vi "Init Error Window.vi"(4 "Window Vertical Size (pixels)":i16=600, 5 "Window Behaviour":T1, 6 "Window Horizontal Size (pixels)":i16=800, 7 "Window Close (X) Button Enabled? (Default = True)":bool=TRUE, 8 "Error In":errorcluster, 9 "Background Colour (Default = 255,255,255)":u32(colorbox)=16777215, 10 "Window Title":string="Modal Dialogue", 11 "VI Refnum":refnum<vi>) -> (0 "Error Out":errorcluster)   [LabVIEW 2016, in "Error Manager.lvlib"]
doc: "This VI configures the Front Panel (the GUI Window) of the VI whose refnum is passed as an argument to the \"VI Refnum\" input (usually, the immediate caller VI)."
uses:
  Error Manager.lvlib
  <vilib>/Utility/miscctls.llb/LVPointTypeDef.ctl
  <vilib>/Utility/miscctls.llb/LVRectTypeDef.ctl
  Settings/Window_Behaviour (enum).ctl
  Settings/Settings.lvclass
panel:
  # "Development\ncontrols/indicators useful for development and testing, but which are not outputs of the VI"
  # "Input\nInputs to the VI"
  # "Output\nOutputs of the VI"
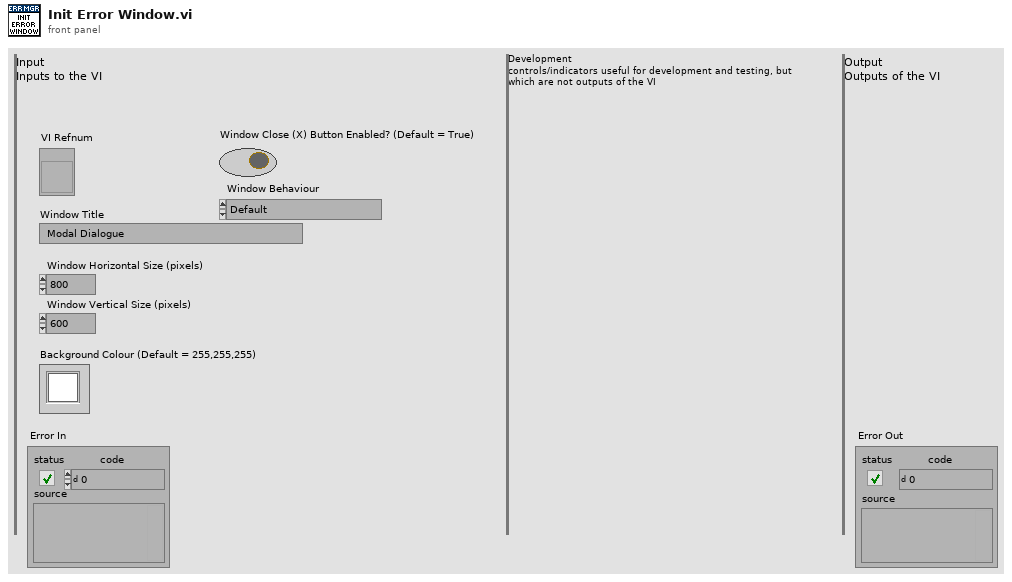
[diagram p1: front panel]
types:
  T1 = typedef "Error Manager.lvlib/Settings.lvclass/Window_Behaviour (enum).ctl" = enum16{"Default", "Floating", "Modal"}
  T2 = enum32{"Invalid", "Standard", "Closed", "Hidden", "Minimized", "Maximized"}
  T3 = typedef "LVRectTypeDef.ctl" = cluster{"Left":i16, "Top":i16, "Right":i16, "Bottom":i16}
  T4 = typedef "LVPointTypeDef.ctl" = cluster{"Horizontal":i16, "Vertical":i16}
  T5 = enum16{"Always On", "Always Off", "Off While Running"}
  T6 = enum32{"Invalid", "Default", "Floating", "Floating/Auto-Hide", "Modal"}
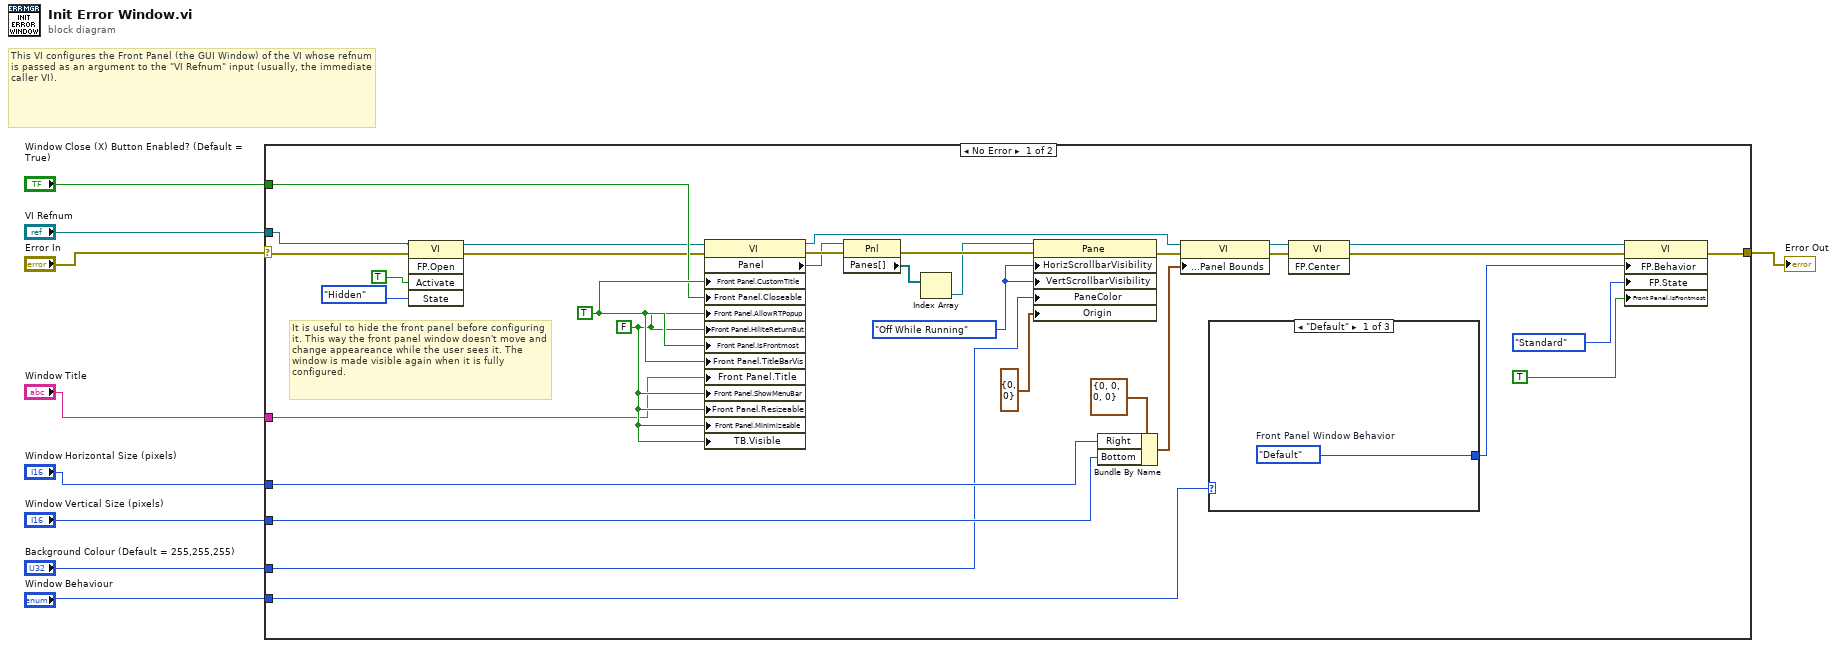
[diagram p0: block diagram]
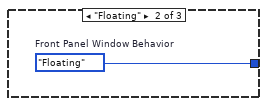
[diagram p2: hidden frame]
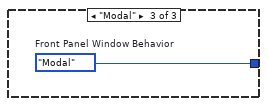
[diagram p3: hidden frame]
diagram:
  # "This VI configures the Front Panel (the GUI Window) of the VI whose refnum is passed as an argument to the \"VI Refnum\" input (usually, the immediate caller VI)."
  n1 = case shown="No Error" "Error In" {
    selector: "Error In" -> [w20 w46]
    tunnel: [w14 w46] -> w8
    tunnel: "VI Refnum" -> [w18 _]
    tunnel: "Window Title" -> [w27 _]
    tunnel: "Window Horizontal Size (pixels)" -> [w26 _]
    tunnel: "Window Vertical Size (pixels)" -> [w25 _]
    tunnel: "Window Close (X) Button Enabled? (Default = True)" -> [w24 _]
    tunnel: "Background Colour (Default = 255,255,255)" -> [w23 _]
    tunnel: "Window Behaviour" -> [w10 _]
    frame No Error {
      w36 = T5."Off While Running" ("Horizontal Scrollbar Visibility")
      w35 = FALSE
      w41 = TRUE
      # "It is useful to hide the front panel before configuring it. This way the front panel window doesn't move and change appeareance while the user sees it. The window is made visible again when it is fully configured."
      n2 = invoke class="VI" method="FP.Open"(reference=w18, error in=w20, "Activate"=TRUE ("Activate?"), "State"=T2."Hidden") -> (reference out=w17:refnum<vi>, error out=w19:errorcluster)  [unwired: 1 in, 3 out]
      n3 = property class="VI"(reference=w17, error in=w19, "Front Panel.CustomTitle"=w41, "Front Panel.Closeable"=w24, "Front Panel.AllowRTPopup"=w35, "Front Panel.HiliteReturnBut"=w35, "Front Panel.IsFrontmost"=w41, "Front Panel.TitleBarVis"=w41, "Front Panel.Title"=w27, "Front Panel.ShowMenuBar"=w35, "Front Panel.Resizeable"=w35, "Front Panel.Minimizeable"=w35, "TB.Visible"=w35) -> (reference out=w31:refnum<vi>, error out=w42:errorcluster, "Panel"=w39:refnum<vi>)
      n4 = property class="Pnl"(reference=w39, error in=w42) -> (error out=w40:errorcluster, "Panes[]"=w38:refnum<vi>[])  [unwired: 1 out]
      n5 = Index Array(array=w38) -> (element=w37:refnum<vi>)  [unwired: 1 in]
      n6 = property class="Pane"(reference=w37, error in=w40, "HorizScrollbarVisibility"=w36, "VertScrollbarVisibility"=w36, "PaneColor"=w23, "Origin"=T4 {"Horizontal"=0, "Vertical"=0}) -> (error out=w33:errorcluster)  [unwired: 1 out]
      n7 = Bundle By Name(cluster=T3 {"Left"=0, "Top"=0, "Right"=0, "Bottom"=0} ("Front Panel Window:Panel Bounds"), "Right"=w26, "Bottom"=w25) -> (w29:T3)
      n8 = property on="Property Node" class="VI"(reference=w31, error in=w33, "Front Panel Window:Panel Bounds"=w29) -> (reference out=w28:refnum<vi>, error out=w32:errorcluster)
      n9 = case shown="\"Default\"" w10 {
        tunnel: [w43 w44 w45] -> w11
        frame "Default" {
          w43 = T6."Default"  # Front Panel Window Behavior
        }
        frame "Floating" {
          w44 = T6."Floating"  # Front Panel Window Behavior
        }
        frame "Modal" {
          w45 = T6."Modal"  # Front Panel Window Behavior
        }
      }
      n10 = invoke class="VI" method="FP.Center"(reference=w28, error in=w32) -> (reference out=w12:refnum<vi>, error out=w13:errorcluster)  [unwired: 1 in, 1 out]
      n11 = property class="VI"(reference=w12, error in=w13, "FP.Behavior"=w11, "FP.State"=T2."Standard" ("Front Panel Window:State"), "Front Panel.IsFrontmost"=TRUE ("Front Panel Window:Is Frontmost")) -> (error out=w14:errorcluster)  [unwired: 1 out]
    }
    frame Error {
    }
  }
  "Error Out" <- w8
